vi "DO Remains.vi"(11 "Array":T1(array[cluster])) -> (0 "Status":string, 1 "DO value":bool[](array[boolean]), 2 "Same DO":T1(array[cluster]), 3 "Remains":T1(array[cluster]))   [LabVIEW 2022 SP3]
uses:
  RT Controls/DO FGV.ctl
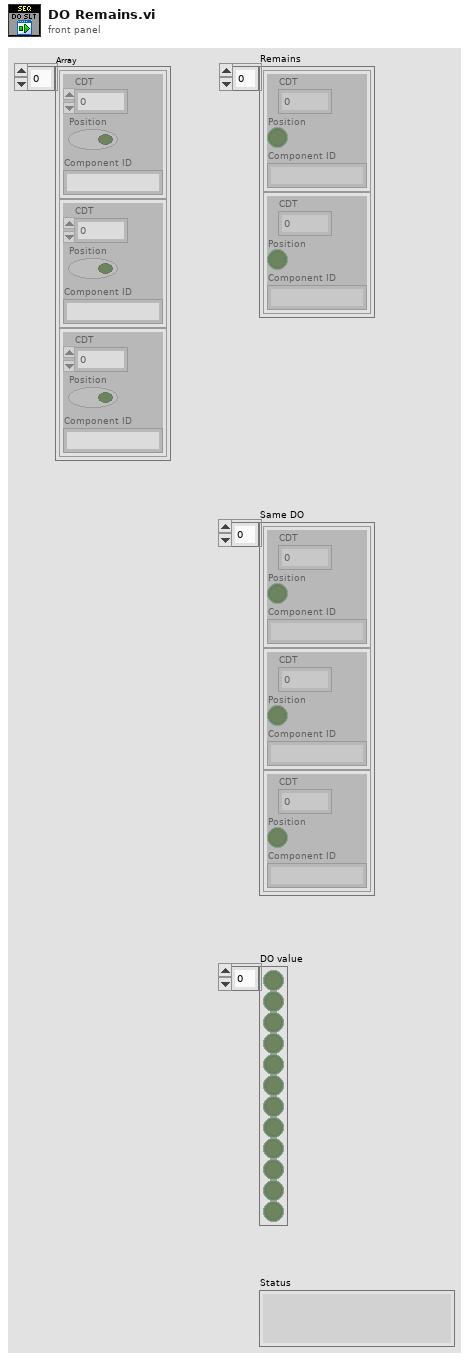
[diagram p1: front panel]
types:
  T1 = cluster{"CDT":dbl, "Position":bool, "Component ID":string}[]
  T2 = typedef "DO FGV.ctl" = enum16{"Read", "Write", "Start time", "init", "Read only"}
  T3 = cluster{"CDT":dbl, "Position":bool, "Component ID":string}
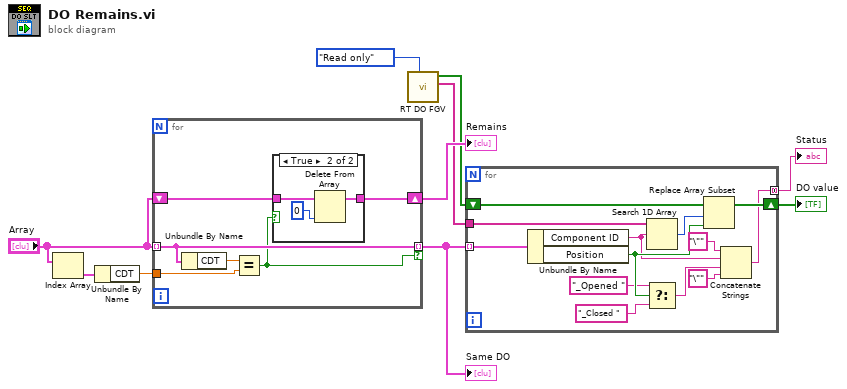
[diagram p0: block diagram]
diagram:
  n1 = Index Array(array="Array") -> (element=w7:T3)  [unwired: 1 in]
  n2 = Unbundle By Name(w7) -> ("CDT"=w9:dbl)
  n3 = for {
    tunnel: "Array" -> [w12] mode=indexing
    shift-right: [w15] -> w10
    shift-left: "Array" -> [w16]
    tunnel: w9 -> [w13]
    tunnel: [w12] -> w6 mode=indexing if=w11
    n4 = Unbundle By Name(w12) -> ("CDT"=w14:dbl)
    n5 = Equal?(x=w14, y=w13) -> (x = y?=w11:bool)
    n6 = case shown="True" w11 {
      tunnel: w16 -> [w17 w20]
      tunnel: [w17 w19] -> w15
      frame False {
      }
      frame True {
        n7 = Delete From Array(array=w20, index=0) -> (array with subset deleted=w19:T1)  [unwired: 1 in, 1 out]
      }
    }
  }
  "Remains" <- w10
  "Same DO" <- w6
  n8 = call "RT DO FGV.vi"("Enum"=DO_FGV."Read only") -> ("DO Names Out"=w2:string[], "DO out"=w3:bool[])  [unwired: 8 in, 1 out]
  n9 = for {
    tunnel: w6 -> [w33] mode=indexing
    tunnel: w2 -> [w29]
    shift-right: [w31] -> w5
    shift-left: w3 -> [w32]
    tunnel: [w23] -> w1 mode=concatenating
    n10 = Unbundle By Name(w33) -> ("Component ID"=w24:string, "Position"=w28:bool)
    n11 = Search 1D Array(1D array=w29, element=w24) -> (index of element=w30:i32)  [unwired: 1 in]
    n12 = Select(t="_Opened ", s=w28, f="_Closed ") -> (s? t:f=w25:string)
    n13 = Replace Array Subset(array=w32, new element=w28, index=w30) -> (w31:bool[])
    n14 = Concatenate Strings("\"" ("string"), w24, w25, "\"" ("string")) -> (w23:string)
  }
  "DO value" <- w5
  "Status" <- w1
